vi "Find Resource by Type (String).vi"(10 "Resource Type":string, 11 "Resources":T2) -> (1 "Index":i32, 2 "Found?":bool, 3 "Resource":T1)   [LabVIEW 2017]
uses:
  Resource Array.ctl
  Resource.ctl
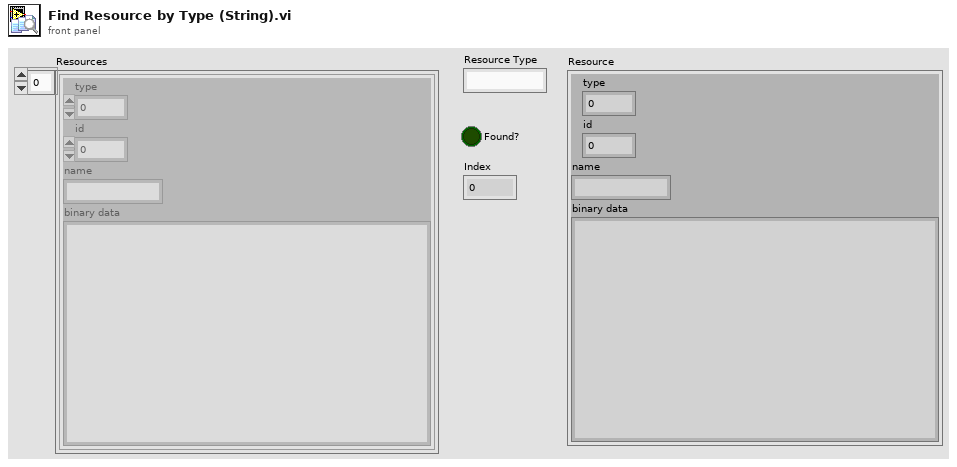
[diagram p1: front panel]
types:
  T1 = typedef "Resource.ctl" = cluster{"type":u32, "id":i32, "name":string, "binary data":string}
  T2 = typedef "Resource Array.ctl" = T1[]
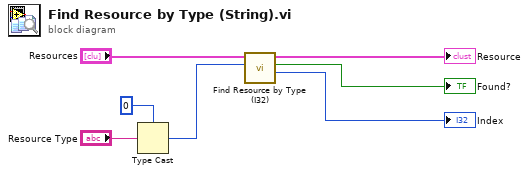
[diagram p0: block diagram]
diagram:
  n1 = Type Cast(type=u32 0 ("Resource Type"), x="Resource Type") -> (*(type *) &x=w4:u32)
  n2 = call "Find Resource by Type (I32).vi"("Resource Type"=w4, "Resources"="Resources") -> ("Index"=→"Index":i32, "Found?"=→"Found?":bool, "Resource"=→"Resource":T1)  [unwired: 7 in]
